vi "IMAQdx Acquisition Template (Simulated FPGA VI).vi"() -> ()   [LabVIEW 2015]
uses:
  <vilib>/rvi/interface/nirviOpenFPGA/nirviOpenFPGA.xnode
  <vilib>/rvi/interface/nirviCloseFPGA/nirviCloseFPGA.xnode
  <vilib>/rvi/interface/nirviMethod/nirviMethod.xnode
  <vilib>/vision/driver/NI_Vision_Acquisition_Software.lvlib
  <resource>/objmgr/imaqdx.rc
  <vilib>/vision/driver/IMAQdx.llb/IMAQdx Acquisition Mode.ctl
  <vilib>/vision/driver/IMAQdx.llb/IMAQdx Buffer Number Mode.ctl
  <vilib>/FPGAPlugInAG/Dynamic/niLvFpga_Run_Dynamic.vi
  <vilib>/rvi/interface/nirviReadWriteControl/nirviReadWriteControl.xnode
  <vilib>/FPGAPlugInAG/Dynamic/niLvFpga_ConfigureFifo_Dynamic.vi
  <vilib>/rvi/errors/niLvFpgaMergeErrorWithErrorCode.vi
  <vilib>/FPGAPlugInAG/Dynamic/niLvFpga_StartFifo_Dynamic.vi
  <vilib>/vision/EDVR.llb/IMAQ ImageToEDVR 2D U8.vi
  <vilib>/FPGA/interface/niFpgaViExecutionMode.ctl
  FPGA Bitfiles/ImageProcessingw_FPGATarget_ImageProcessingw_dnnRZNa3Cr0.lvbitx
  Image Processing with Vision Assistant (FPGA).vi
  <vilib>/rvi/interface/common/dynamic/niFpgaDynamicGetExecutionMode.vi
  <vilib>/rvi/interface/Simulation/niFpgaSimulationCallBeginRW.vi
  <vilib>/rvi/errors/niLvFpgaAdjustHostInterfaceError.vi
  <vilib>/FPGAPlugInAG/Dynamic/niLvFpga_WriteFifo_Dynamic.vi
  <vilib>/FPGAPlugInAG/Dynamic/niLvFpga_ReadFifo_Dynamic.vi
  <vilib>/FPGAPlugInAG/Dynamic/niLvFpga_Close_Dynamic.vi
  <vilib>/userdefined/High Color/IMAQdx.ctl
panel:
  out "Processed Image Count":i32
  in  "Camera":T1
  out "Error Out":errorcluster
  out "Image":T2(plugin-control)
  in  "Stop":bool
  # "Overview: Demonstrates how to acquire an image from a camera using the IMAQdx API and simulate the processing of the image on the FPGA.  This VI is only intended to be used when the FPGA Target is configured to be in the \"Simulation (Simulated I/O)\" Execution Mode.  Simulation is only supported in the \"My Computer\" execution context (i.e. not on a Real-Time target).\nRequirements:\n- LabVIEW FPGA\n- Vision Acquisition Software\n- Vision Development Module\nInstructions:\n1. Select a Camera\n2. Run the VI."
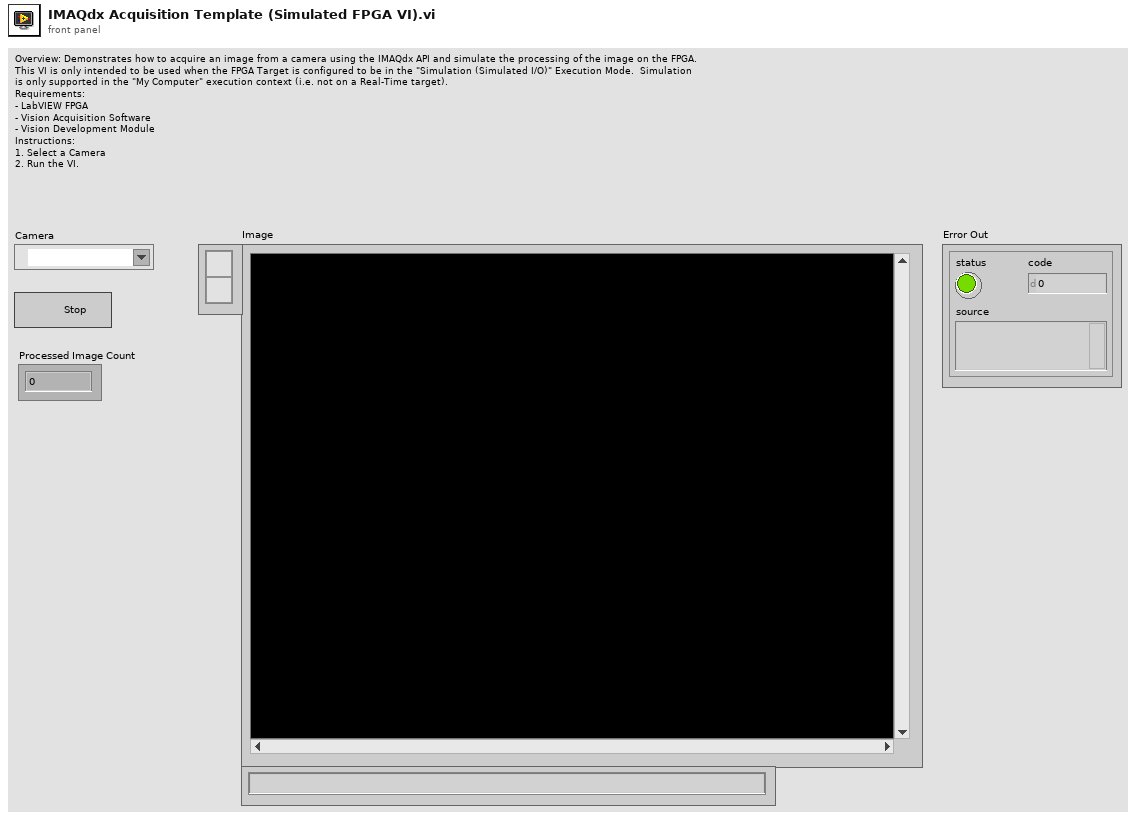
[diagram p1: front panel]
types:
  T1 = typedef "IMAQdx.ctl" = refnum<k21>
  T2 = typedef "IMAQ Image.ctl" = refnum<image>
  T3 = typedef "niFpgaViExecutionMode.ctl" = enum16{"FPGA Target", "Simulation (Simulated I/O)", "Simulation (Real I/O)", "Third-Party Simulation"}
  T4 = typedef "Image Type" = u32
  T5 = typedef "NI_Vision_Acquisition_Software.lvlib/IMAQdx Acquisition Mode.ctl" = enum32{"One Shot", "Continuous"}
  T6 = typedef "NI_Vision_Acquisition_Software.lvlib/IMAQdx Buffer Number Mode.ctl" = enum32{"Next", "Last", "Buffer Number", "Every", "Last New"}
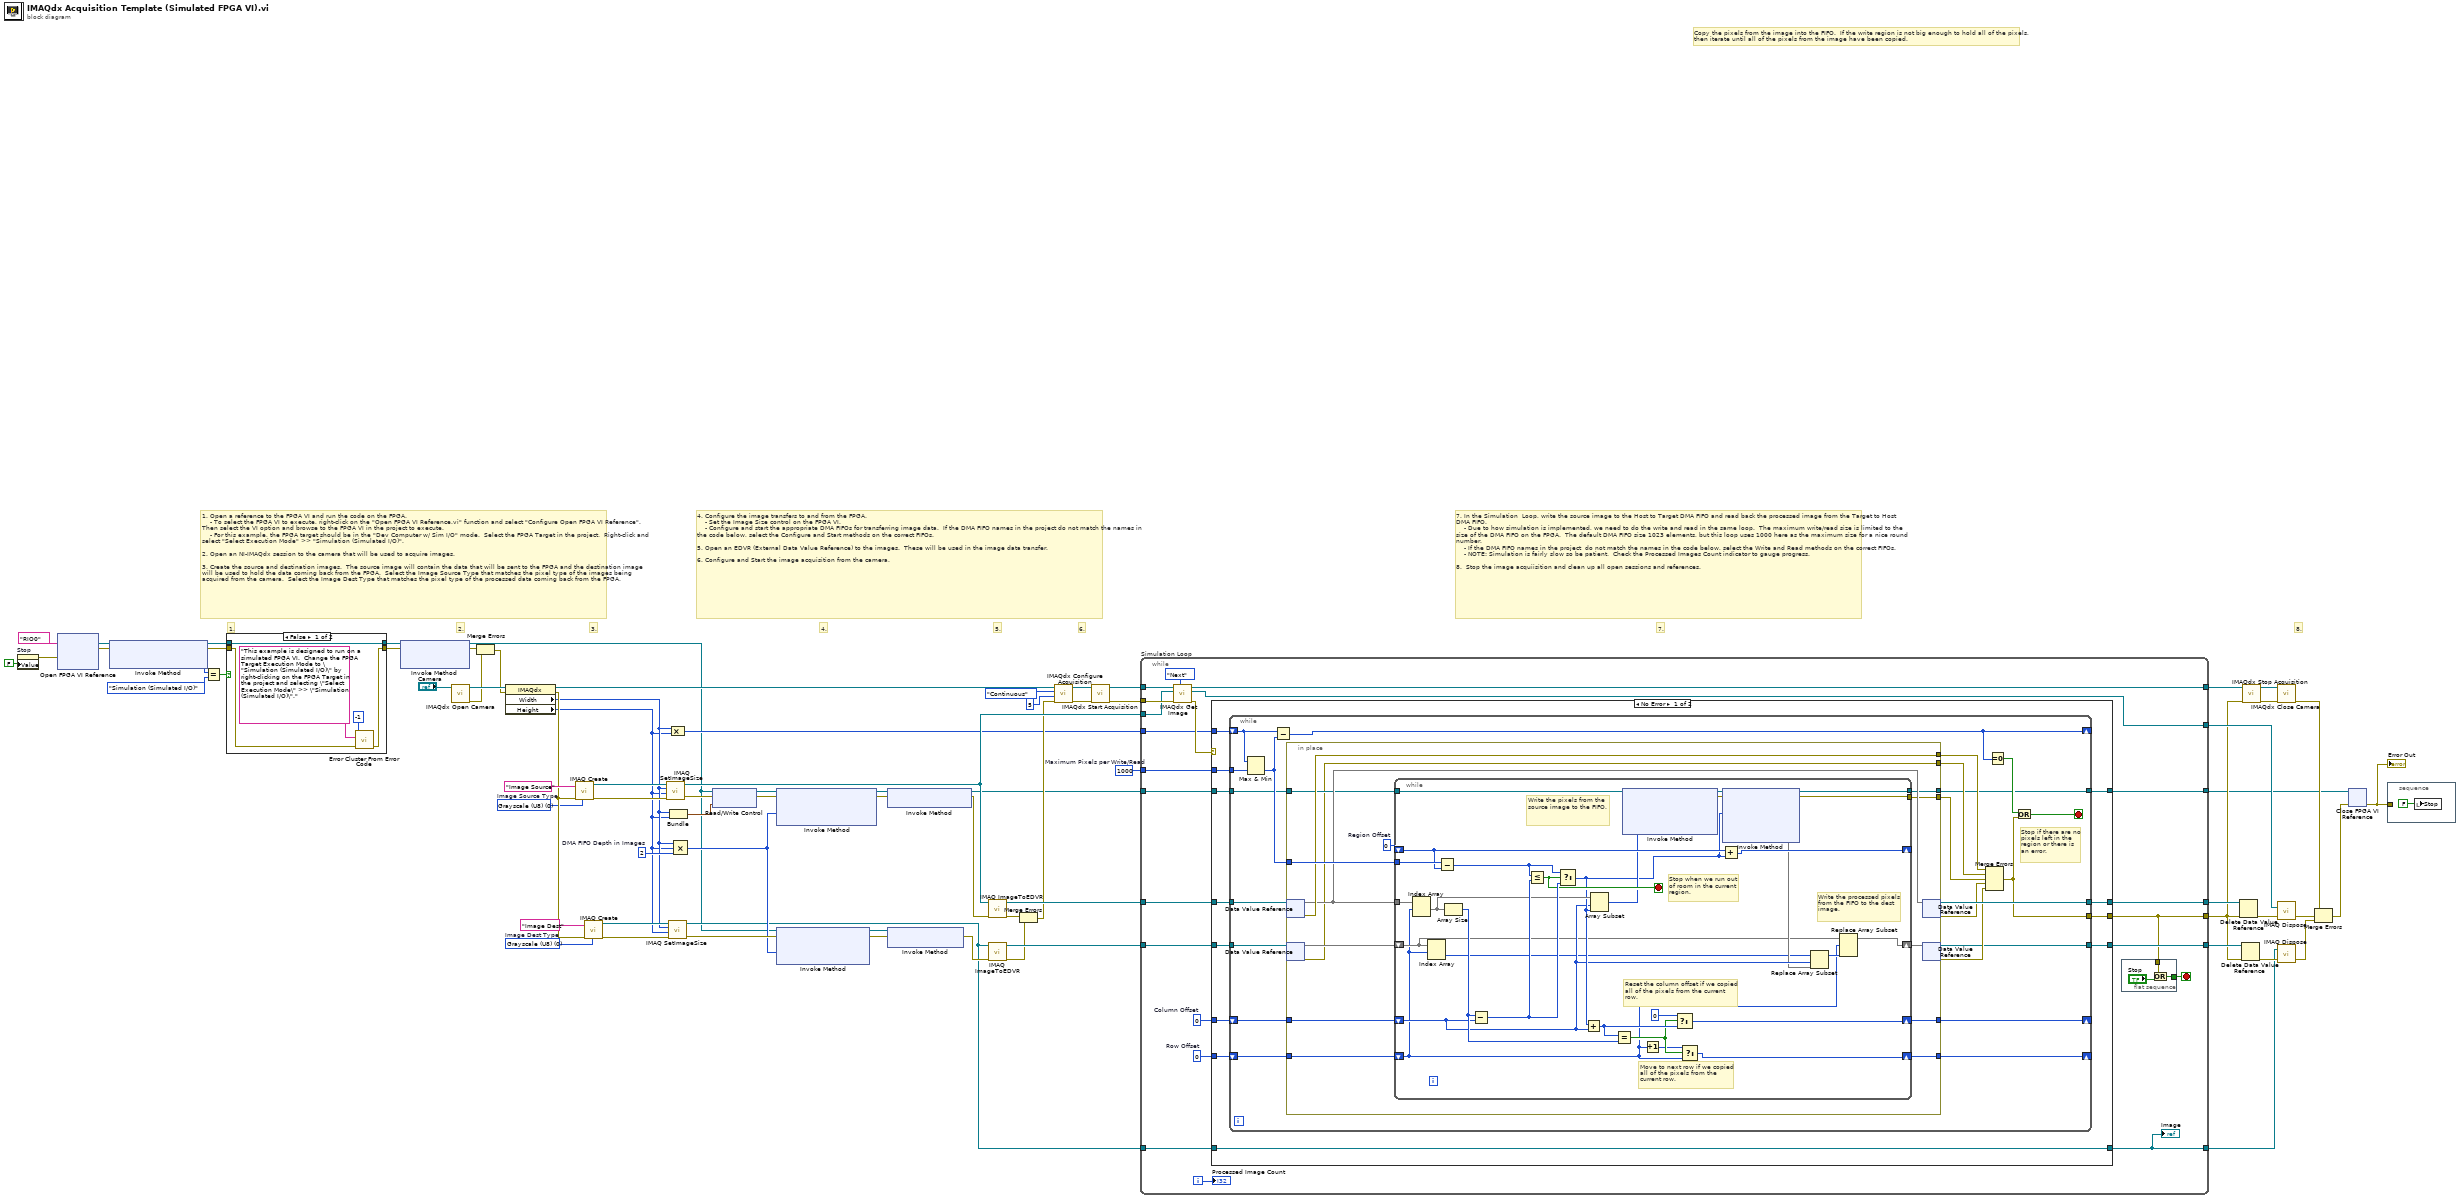
[diagram p0: block diagram]
diagram:
  w12 = u32 1000  # Maximum Pixels per Write/Read
  w43 = u32 2  # DMA FIFO Depth in Images
  w52 = T4 0 items=["Grayscale (U8)", "Grayscale (I16)", "Grayscale (SGL)", "Complex (CSG)", "RGB (U32)", "HSL (U32)", "RGB (U64)", "Grayscale (U16)"]  # Image Dest Type
  w53 = T4 0 items=["Grayscale (U8)", "Grayscale (I16)", "Grayscale (SGL)", "Complex (CSG)", "RGB (U32)", "HSL (U32)", "RGB (U64)", "Grayscale (U16)"]  # Image Source Type
  # "7. In the Simulation  Loop, write the source image to the Host to Target DMA FIFO and read back the processed image from the Target to Host DMA FIFO.  \n    - Due to how simulation is implemented, we need to do the write and read in the same loop.  The maximum write/read size is limited to the size of the DMA FIFO on the FPGA.  The default DMA FIFO size 1023 elements, but this loop uses 1000 here as the maximum size for a nice round number.\n    - If the DMA FIFO names in the project  do not match the names in the code below, select the Write and Read methods on the correct FIFOs. \n    - NOTE: Simulation is fairly slow so be patient.  Check the Processed Images Count indicator to gauge progress.\n\n8.  Stop the image acquiisition and clean up all open sessions and references."
  # "4. Configure the image transfers to and from the FPGA.  \n    - Set the Image Size control on the FPGA VI. \n    - Configure and start the appropriate DMA FIFOs for transferring image data.  If the DMA FIFO names in the project do not match the names in the code below, select the Configure and Start methods on the correct FIFOs. \n\n5. Open an EDVR (External Data Value Reference) to the images.  These will be used in the image data transfer.\n\n6. Configure and Start the image acquisition from the camera."
  # "Copy the pixels from the image into the FIFO.  If the write region is not big enough to hold all of the pixels,\nthen iterate until all of the pixels from the image have been copied."
  # "1. Open a reference to the FPGA VI and run the code on the FPGA.\n    - To select the FPGA VI to execute, right-click on the \"Open FPGA VI Reference.vi\" function and select \"Configure Open FPGA VI Reference\".  Then select the VI option and browse to the FPGA VI in the project to execute.\n    - For this example, the FPGA target should be in the \"Dev Computer w/ Sim I/O\" mode.  Select the FPGA Target in the project.  Right-click and select \"Select Execution Mode\" >> \"Simulation (Simulated I/O)\".\n\n2. Open an NI-IMAQdx session to the camera that will be used to acquire images.\n\n3. Create the source and destination images.  The source image will contain the data that will be sent to the FPGA and the destination image will be used to hold the data coming back from the FPGA.  Select the Image Source Type that matches the pixel type of the images being acquired from the camera.  Select the Image Dest Type that matches the pixel type of the processed data coming back from the FPGA."
  # "8."
  # "7."
  # "6."
  # "5."
  # "4."
  # "3."
  # "2."
  # "1."
  n1 = property on="Stop" class="Bool (strict)"("Value"=FALSE ("Stop")) -> (error out=w3:errorcluster)  [unwired: 2 in, 1 out]
  n2 = xnode "Open FPGA VI Reference"("error in"=w3, "resource name"=tag "RIO0") -> ("FPGA VI Reference Out"=w11:refnum<k20>, "error out"=w10:errorcluster)
  n3 = xnode "Invoke Method"("FPGA VI Reference In"=w11, "error in"=w10) -> ("FPGA VI Reference Out"=w6:refnum<k20>, "error out"=w5:errorcluster, "FPGA VI Execution Mode"=w9:T3)
  n4 = Equal?(x=w9, y=niFpgaViExecutionMode."Simulation (Simulated I/O)" ("FPGA VI Execution Mode")) -> (x = y?=w7:bool)
  n5 = case shown="False" w7 {
    tunnel: [w80 w82] -> w2
    tunnel: w6 -> [w80 w82]
    tunnel: w5 -> [w76 w81]
    tunnel: [w79 w81] -> w1
    frame False {
      n6 = call <vilib>:"Error Cluster From Error Code.vi"("error in (no error)"=w76, "error message (\"\")"="This example is designed to run on a simulated FPGA VI.  Change the FPGA Target Execution Mode to \"Simulation (Simulated I/O)\" by right-clicking on the FPGA Target in the project and selecting \"Select Execution Mode\" >> \"Simulation (Simulated I/O)\"." ("error message (\"\")"), "error code (0)"=-1) -> ("error out"=w79:errorcluster)  [unwired: 6 in]
    }
    frame True {
    }
  }
  n7 = xnode "Invoke Method"("FPGA VI Reference In"=w2, "error in"=w1) -> ("FPGA VI Reference Out"=w14:refnum<k20>, "error out"=w71:errorcluster)  [unwired: 1 in]
  n8 = call <vilib>:"IMAQdx Open Camera.vi"("Session In"="Camera") -> ("error out"=w58:errorcluster, "Session Out"=w59:T1)  [unwired: 9 in]
  n9 = Merge Errors(w71, w58) -> (w57:errorcluster)
  n10 = property class="IMAQdx"(reference=w59, error in=w57) -> (reference out=w66:T1, error out=w54:errorcluster, "Width"=w19:u32, "Height"=w18:u32)
  n11 = call "IMAQ Create"("Image Name"="Image Source", "Image Type"=w53, "error in (no error)"=w54) -> ("New Image"=w50:T2, "error out"=w51:errorcluster)  [unwired: 2 in]
  n12 = call "IMAQ Create"("Image Name"="Image Dest", "Image Type"=w52, "error in (no error)"=w54) -> ("New Image"=w49:T2, "error out"=w48:errorcluster)  [unwired: 2 in]
  n13 = call "IMAQ SetImageSize"("error in (no error)"=w51, "Y Resolution"=w18, "X Resolution"=w19, "Image"=w50) -> ("error out"=w47:errorcluster, "Image Out"=w33:T2)  [unwired: 1 in]
  n14 = call "IMAQ SetImageSize"("error in (no error)"=w48, "Y Resolution"=w18, "X Resolution"=w19, "Image"=w49) -> ("error out"=w38:errorcluster, "Image Out"=w16:T2)  [unwired: 1 in]
  n15 = Bundle("Width"=w19, "Height"=w18) -> (w46:cluster{"Width":u32, "Height":u32})  [unwired: 1 in]
  n16 = Compound Arithmetic op=MULTIPLY(w19, w18) -> (w17:u32)
  n17 = Compound Arithmetic op=MULTIPLY(w19, w18, w43) -> (w37:u32)
  n18 = xnode "Read/Write Control"("FPGA VI Reference In"=w14, "error in"=w47, "Image Size"=w46) -> ("FPGA VI Reference Out"=w44:refnum<k20>, "error out"=w45:errorcluster)
  n19 = xnode "Invoke Method"("FPGA VI Reference In"=w44, "error in"=w45, "Requested Depth"=w37) -> ("FPGA VI Reference Out"=w42:refnum<k20>, "error out"=w41:errorcluster)  [unwired: 1 out]
  n20 = xnode "Invoke Method"("FPGA VI Reference In"=w14, "error in"=w38, "Requested Depth"=w37) -> ("FPGA VI Reference Out"=w40:refnum<k20>, "error out"=w39:errorcluster)  [unwired: 1 out]
  n21 = xnode "Invoke Method"("FPGA VI Reference In"=w42, "error in"=w41) -> ("FPGA VI Reference Out"=w20:refnum<k20>, "error out"=w34:errorcluster)
  n22 = xnode "Invoke Method"("FPGA VI Reference In"=w40, "error in"=w39) -> ("error out"=w31:errorcluster)  [unwired: 1 out]
  n23 = call-poly <vilib>:"IMAQ ImageToEDVR.vi"("error in (no error)"=w34, "Image"=w33) -> ("error out"=w32:errorcluster, "EDVR 2D U8"=w35:refnum<data-value>)  [unwired: 7 in, 1 out]
  n24 = call-poly <vilib>:"IMAQ ImageToEDVR.vi"("error in (no error)"=w31, "Image"=w16) -> ("error out"=w28:errorcluster, "EDVR 2D U8"=w30:refnum<data-value>)  [unwired: 7 in, 1 out]
  n25 = Merge Errors(w32, w28) -> (w29:errorcluster)
  n26 = call <vilib>:"IMAQdx Configure Acquisition.vi"("error in"=w29, "Number of Buffers"=u32 5, "Continuous?"=IMAQdx_Acquisition_Mode."Continuous", "Session In"=w66) -> ("error out"=w69:errorcluster, "Session Out"=w70:T1)  [unwired: 6 in]
  n27 = call <vilib>:"IMAQdx Start Acquisition.vi"("error in"=w69, "Session In"=w70) -> ("error out"=w62:errorcluster, "Session Out"=w65:T1)  [unwired: 8 in]
  n28 = while "Simulation Loop" {
    tunnel: [w87] -> w24
    tunnel: w33 -> [w99]
    tunnel: w20 -> [w94]
    tunnel: w65 -> [w102]
    tunnel: [w101] -> w61
    tunnel: w62 -> [w100]
    tunnel: [w98] -> w36
    tunnel: w35 -> [w96]
    tunnel: w30 -> [w97]
    tunnel: w16 -> [w90]
    tunnel: [w88] -> w27
    tunnel: [w89] -> w25
    tunnel: w17 -> [w93]
    tunnel: [w85] -> w15
    tunnel: [w84] -> w13
    tunnel: w12 -> [w83]
    i -> [w86]
    stop <- w104 stop-if-true
    w91 = u32 0  # Row Offset
    w92 = u32 0  # Column Offset
    n29 = call <vilib>:"IMAQdx Get Image.vi"("Buffer Number Mode (Next)"=IMAQdx_Buffer_Number_Mode."Next", "error in"=w100, "Image In"=w99, "Session In"=w102) -> ("error out"=w95:errorcluster, "Image Out"=w98:T2, "Session Out"=w101:T1)  [unwired: 4 in, 1 out]
    n30 = case shown="No Error" w95 {
      selector: w95 -> [_ w186]
      tunnel: w93 -> [w116 _]
      tunnel: w96 -> [w115 w185]
      tunnel: w92 -> [w114 _]
      tunnel: w91 -> [w113 _]
      tunnel: w94 -> [w112 w182]
      tunnel: [w111 w186] -> w87
      tunnel: [w110 w185] -> w88
      tunnel: w83 -> [w109 _]
      tunnel: w97 -> [w108 w183]
      tunnel: w90 -> [w107 w184]
      tunnel: [w107 w184] -> w85
      tunnel: [w106 w183] -> w89
      tunnel: [w105 w182] -> w84
      frame No Error {
        n31 = while {
          shift-right: [w132] -> _
          shift-left: w116 -> [w128]
          tunnel: w115 -> [w138]
          shift-right: [w134] -> _
          shift-left: w114 -> [w136]
          shift-right: [w137] -> _
          shift-left: w113 -> [w135]
          tunnel: w112 -> [w125]
          tunnel: [w133] -> w110
          tunnel: [w130] -> w111
          tunnel: w109 -> [w127]
          tunnel: w108 -> [w124]
          tunnel: [w118] -> w106
          tunnel: [w117] -> w105
          stop <- w131 stop-if-true
          # "Stop if there are no\npixels left in the \nregion or there is\nan error."
          n32 = Max & Min(x=w128, y=w127) -> (min(x,y)=w126:u32)  [unwired: 1 out]
          n33 = Subtract(x=w128, y=w126) -> (x-y=w132:u32)
          n34 = in-place {
            in-place-border: w126 -> [w150]
            in-place-border: [w152] -> w137
            in-place-border: w136 -> [w149]
            in-place-border: w135 -> [w146]
            in-place-border: [w148] -> w134
            in-place-border: [w147] -> w121
            in-place-border: w125 -> [w144]
            in-place-border: [w141] -> w120
            in-place-border: [w140] -> w119
            in-place-border: [w139] -> w117
            w151 = u32 0  # Region Offset
            n35 = in-place-dvr #1(w138) -> (w145:u8[][], w147:errorcluster)
            n36 = in-place-dvr #2(w124) -> (w143:u8[][], w141:errorcluster)
            n37 = while {
              tunnel: w145 -> [w168]
              shift-right: [w179] -> _
              shift-left: w151 -> [w178]
              tunnel: w150 -> [w181]
              shift-right: [w173] -> w148
              shift-left: w149 -> [w160]
              shift-right: [w170] -> w152
              shift-left: w146 -> [w154]
              tunnel: w144 -> [w166]
              shift-right: [w156] -> w142
              shift-left: w143 -> [w157]
              tunnel: [w155] -> w140
              tunnel: [w153] -> w139
              stop <- w169 stop-if-true
              # "Write the processed pixels from the FIFO to the dest image."
              # "Stop when we run out\nof room in the current\nregion."
              # "Write the pixels from the source image to the FIFO."
              # "Reset the column offset if we copied\nall of the pixels from the current\nrow."
              # "Move to next row if we copied\nall of the pixels from the\ncurrent row."
              n38 = Index Array(array=w168, index (row)=w154) -> (element=w167:u8[])  [unwired: 1 in]
              n39 = Index Array(array=w157, index (row)=w154) -> (element=w158:u8[])  [unwired: 1 in]
              n40 = Subtract(x=w181, y=w178) -> (x-y=w180:u32)
              n41 = Array Size(array=w167) -> (size(s)=w177:i32)
              n42 = Subtract(x=w177, y=w160) -> (x-y=w176:u32)
              n43 = Less Or Equal?(x=w180, y=w176) -> (x <= y?=w169:bool)
              n44 = Select(t=w180, s=w169, f=w176) -> (s? t:f=w162:u32)
              n45 = Add(x=w162, y=w160) -> (x+y=w174:u32)
              n46 = Array Subset(array=w167, index=w160, length=w162) -> (w165:u8[])
              n47 = Equal?(x=w174, y=w177) -> (x = y?=w172:bool)
              n48 = xnode "Invoke Method"("FPGA VI Reference In"=w166, "Data"=w165) -> ("FPGA VI Reference Out"=w164:refnum<k20>, "error out"=w163:errorcluster)  [unwired: 2 in, 1 out]
              n49 = Increment(x=w154) -> (x+1=w171:u32)
              n50 = Select(t=u32 0 ("Elements In Region"), s=w172, f=w174) -> (s? t:f=w173:u32)
              n51 = Select(t=w171, s=w172, f=w154) -> (s? t:f=w170:u32)
              n52 = xnode "Invoke Method"("FPGA VI Reference In"=w164, "error in"=w163, "Number of Elements"=w162) -> ("FPGA VI Reference Out"=w153:refnum<k20>, "error out"=w155:errorcluster, "Data"=w159:void[])  [unwired: 1 in, 1 out]
              n53 = Add(x=w178, y=w162) -> (x+y=w179:u32)
              n54 = Replace Array Subset(array=w158, new element=w159, index=w160) -> (w161:u8[])
              n55 = Replace Array Subset(array=w157, new element=w161, index (row)=w154) -> (w156:u8[][])  [unwired: 1 in]
            }
            n56 = in-place-dvr #1(w145) -> (w133:refnum<data-value>, w123:errorcluster)
            n57 = in-place-dvr #2(w142) -> (w118:refnum<data-value>, w122:errorcluster)
          }
          n58 = Merge Errors(w121, w120, w119, w123, w122) -> (w130:errorcluster)
          n59 = Equal To 0?(x=w132) -> (x = 0?=w129:bool)
          n60 = Or(x=w129, y=w130) -> (x .or. y?=w131:bool)
        }
      }
      frame Error {
      }
    }
    "Image" <- w85
    n61 = flat-sequence {
      tunnel: [w188] -> w104
      tunnel: w87 -> [w187]
      frame #0 {
        n62 = Or(x=w187, y="Stop") -> (x .or. y?=w188:bool)
      }
    }
    "Processed Image Count" <- w86
  }
  n63 = Delete Data Value Reference(data value reference=w27, error in=w24) -> (error out=w26:errorcluster)  [unwired: 1 out]
  n64 = Delete Data Value Reference(data value reference=w25, error in=w24) -> (error out=w23:errorcluster)  [unwired: 1 out]
  n65 = call <vilib>:"IMAQdx Stop Acquisition.vi"("error in"=w24, "Session In"=w61) -> ("error out"=w63:errorcluster, "Session Out"=w64:T1)  [unwired: 8 in]
  n66 = call <vilib>:"IMAQdx Close Camera.vi"("error in"=w63, "Session In"=w64) -> ("error out"=w60:errorcluster)  [unwired: 9 in]
  n67 = call "IMAQ Dispose"("Image"=w36, "error in (no error)"=w26) -> ("error out"=w21:errorcluster)  [unwired: 4 in]
  n68 = call "IMAQ Dispose"("Image"=w15, "error in (no error)"=w23) -> ("error out"=w22:errorcluster)  [unwired: 4 in]
  n69 = Merge Errors(w60, w21, w22) -> (w56:errorcluster)
  n70 = xnode "Close FPGA VI Reference"("FPGA VI Reference In"=w13, "error in"=w56) -> ("error out"=w55:errorcluster)
  "Error Out" <- w55
  n71 = stacked-sequence {
    tunnel: w55 -> [_]
    frame #0 {
      n72 = local write "Stop"(FALSE ("Stop")) -> ()
    }
  }
